vi "Rotation2d_Plus.vi"(9 "other ROTATION":T1 {"SIN" format="%13.4f"; "COS" format="%13.4f"; "VALUE" format="%13.4f"}, 11 "in ROTATION":T1 {"SIN" format="%13.4f"; "COS" format="%13.4f"; "VALUE" format="%13.4f"}) -> (3 "out ROTATION":T1 {"SIN" format="%13.4f"; "COS" format="%13.4f"; "VALUE" format="%13.4f"})   [LabVIEW 2019, in "Trajectory_Library.lvlib"]
doc: "Adds two rotations together, with the result being bounded between -pi and pi.\n\nFor example, Rotation2d.fromDegrees(30) + Rotation2d.fromDegrees(60) = Rotation2d{-pi/2}\n\nThis function is the same as RotateBy.\n\nParameters:\n\n - IN ROTATION - This rotation data structure\n - OTHER ROTATION - The rotation to add.\n\nReturns:\n- OUT ROTATION - The sum of the two rotations."
uses:
  Trajectory_Library.lvlib
  TypeDef/ROTATION2D.ctl
  Rotation2d_CreateXY.vi
  Util_CalcDist.vi
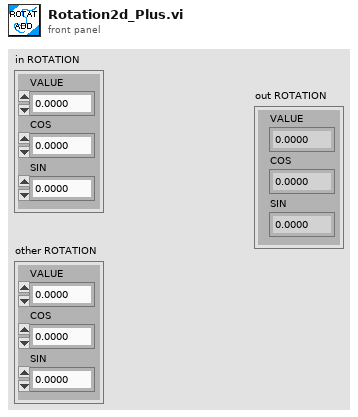
[diagram p1: front panel]
types:
  T1 = typedef "Trajectory_Library.lvlib/ROTATION2D.ctl" = cluster{"VALUE":dbl, "COS":dbl, "SIN":dbl}
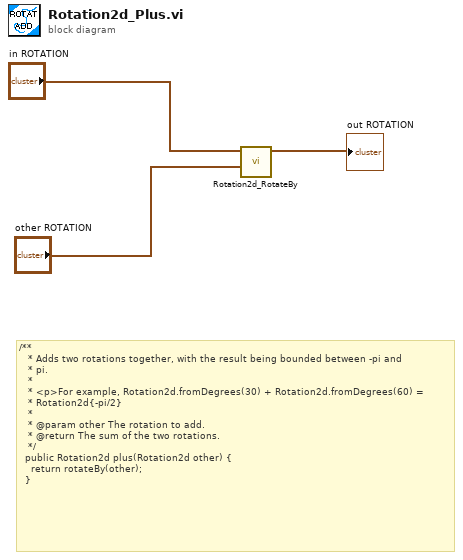
[diagram p0: block diagram]
diagram:
  # "/**\n   * Adds two rotations together, with the result being bounded between -pi and\n   * pi.\n   *\n   * <p>For example, Rotation2d.fromDegrees(30) + Rotation2d.fromDegrees(60) =\n   * Rotation2d{-pi/2}\n   *\n   * @param other The rotation to add.\n   * @return The sum of the two rotations.\n   */\n  public Rotation2d plus(Rotation2d other) {\n    return rotateBy(other);\n  }"
  n1 = call "Rotation2d_RotateBy.vi"("other Rotation"="other ROTATION", "in ROTATION"="in ROTATION") -> ("out ROTATION"=→"out ROTATION":T1)  [unwired: 9 in]
